vi "com VISA_atlas (sub VI).vi"(0 "Sensor":string(combo)="Temp", 1 "entrée d'erreur (pas d'erreur)":errorcluster) -> (2 "Output cluster":T1, 3 "Com found ?":bool)   [LabVIEW 2016]
doc: "Looks for the COM port corresponding to the necessary sensor. For Atlas sensor, sends a Information command (I \\r) and reads the response. Also determines the message size (in bytes) of a typical reading (with a 'R \\r' command)"
uses:
  Visa com cluster def (subVI).ctl
  <vilib>/Instr/_visa.llb/VISA Find Search Mode.ctl
  <vilib>/Instr/_visa.llb/VISA Set IO Buffer Mask.ctl
  <vilib>/Instr/_visa.llb/VISA Flush IO Buffer Mask.ctl
  <vilib>/Instr/_visa.llb/VISA Configure Serial Port (Instr).vi
  <vilib>/regexp/Match Regular Expression.xnode
panel:
  out "Reponse VISA":string
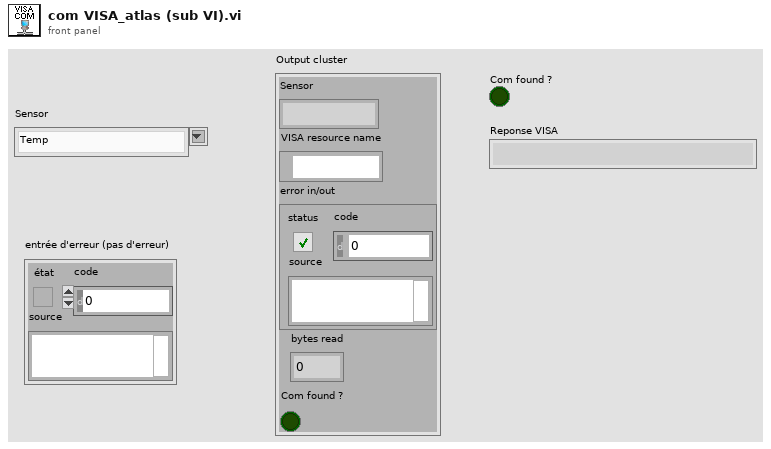
[diagram p1: front panel]
types:
  T1 = typedef "Visa com cluster def (subVI).ctl" = cluster{"Sensor":string, "VISA resource name":refnum<visa-resource-name>, "error in/out":errorcluster, "bytes read":u32, "Com found ?":bool}
  T2 = typedef "VISA Find Search Mode.ctl" = u32
  T3 = cluster{"baud rate":u32, "data bits":u16, "parity":enum16{"None", "Odd", "Even", "Mark", "Space"}, "stop bits":u16, "flow control":u16}
  T4 = typedef "VISA Flush IO Buffer Mask.ctl" = u16
  T5 = typedef "VISA Set IO Buffer Mask.ctl" = u16
  T6 = cluster{"Sensor":string, "VISA resource name out":refnum<visa-resource-name>, "error out":errorcluster, "bytes read":u32, bool}
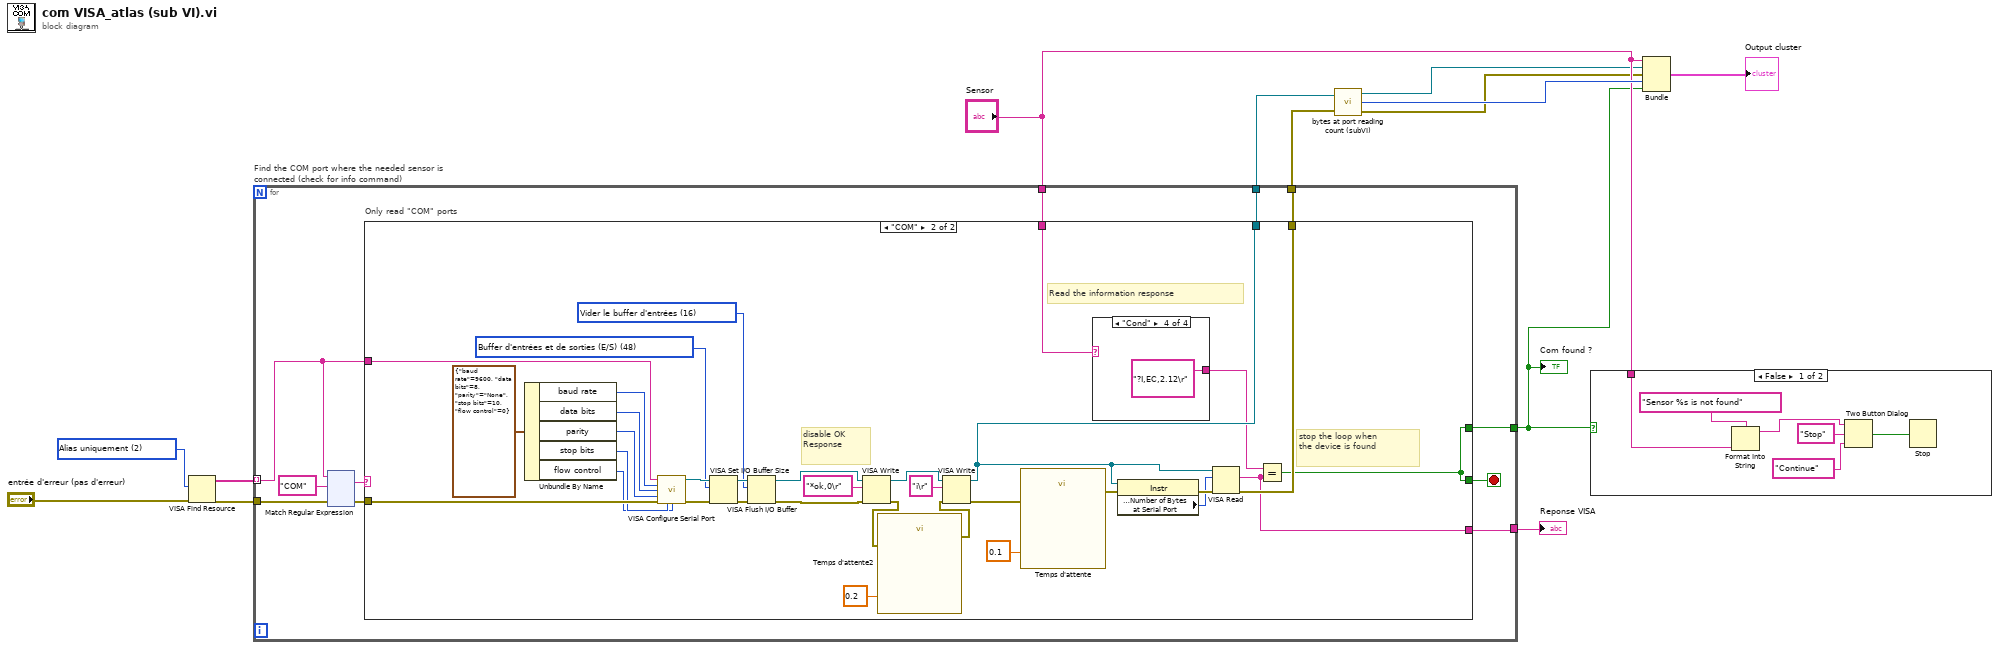
[diagram p0: block diagram]
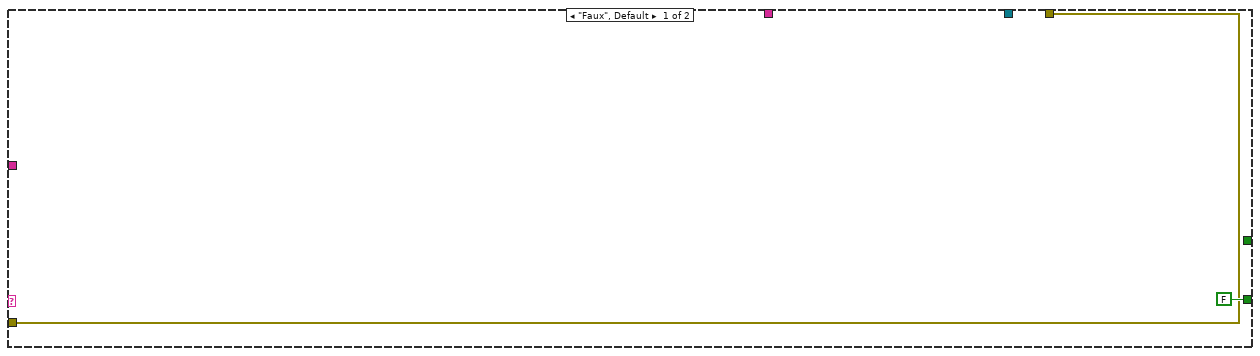
[diagram p3: hidden frame]
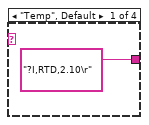
[diagram p4: hidden frame]
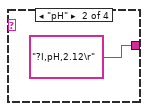
[diagram p5: hidden frame]
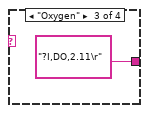
[diagram p6: hidden frame]
diagram:
  w10 = T2 2 items=["Noms canoniques uniquement"=0, "Alias uniquement"=2, "Inclure les alias correspondants"=3, "Inclure tous les alias"=4] ("Search Mode")
  n1 = VISA Find Resource(8:"entrée d'erreur (pas d'erreur)", 10:w10) -> (0:w13:errorcluster, 3:w11:string[])  [unwired: 1 in, 1 out]
  n2 = for "Find the COM port where the needed sensor is connected (check for info command)" {
    tunnel: w11 -> [w22] mode=indexing
    tunnel: [w20] -> w7
    tunnel: [w19] -> w9
    tunnel: [w18] -> w4
    tunnel: w13 -> [w17]
    tunnel: [w15] -> w8
    tunnel: "Sensor" -> [w14]
    stop <- w21 stop-if-true
    n3 = xnode "Match Regular Expression"("chaîne en entrée"=w22, "expression régulière"="COM", "entrée d'erreur"=w17) -> ("toute l'expression"=w23:string, "sortie d'erreur"=w16:errorcluster)  [unwired: 3 in, 3 out]
    n4 = case "Only read \"COM\" ports" shown="\"COM\"" w23 {
      tunnel: w22 -> [_ w50]
      tunnel: [FALSE w47] -> w21
      tunnel: [w25 w49] -> w20
      tunnel: [_ w48] -> w19
      tunnel: [_ w47] -> w18
      tunnel: w16 -> [w25 w46]
      tunnel: [_ w45] -> w15
      tunnel: w14 -> [_ w27]
      frame "Faux", Default {
      }
      frame "COM" {
        w42 = T4 16 items=["Vider le buffer d'entrées"=16, "Écrire le buffer de sorties sur le périphérique"=32, "Vider le buffer d'entrées (Pas d'E/S)"=64, "Vider le buffer de sorties"=128] ("Mask")
        w57 = T5 48 items=["Buffer d'entrées (E/S)"=16, "Buffer de sorties (E/S)"=32, "Buffer d'entrées et de sorties (E/S)"=48] ("Mask")
        # "disable OK\nResponse"
        # "Read the information response"
        # "stop the loop when \nthe device is found"
        n5 = Unbundle By Name(T3 {"baud rate"=9600, "data bits"=8, "parity"=enum."None", "stop bits"=10, "flow control"=0} ("Serial Settings")) -> ("baud rate"=w40:u32, "data bits"=w39:u16, "parity"=w38:enum16{"None", "Odd", "Even", "Mark", "Space"}, "stop bits"=w37:u16, "flow control"=w36:u16)
        n6 = call-poly "VISA Configure Serial Port"("VISA resource name"=w50, "baud rate (9600)"=w40, "data bits (8)"=w39, "parity (0:none)"=w38, "error in (no error)"=w46, "stop bits (10: 1 bit)"=w37, "flow control (0:none)"=w36) -> ("VISA resource name out"=w58:refnum<visa-resource-name>, "error out"=w59:errorcluster)  [unwired: 7 in]
        n7 = VISA Set I/O Buffer Size(VISA resource name=w58, mask (16)=w57, error in (no error)=w59) -> (VISA resource name out=w44:refnum<visa-resource-name>, error out=w43:errorcluster)  [unwired: 1 in]
        n8 = VISA Flush I/O Buffer(VISA resource name=w44, mask (16)=w42, error in (no error)=w43) -> (VISA resource name out=w32:refnum<visa-resource-name>, error out=w33:errorcluster)
        n9 = VISA Write(VISA resource name=w32, write buffer="*ok,0\r" ("buffer d'écriture"), error in (no error)=w33) -> (VISA resource name out=w31:refnum<visa-resource-name>, error out=w29:errorcluster)  [unwired: 1 out]
        n10 = call "Temps d'attente2"("error in (no error)"=w29, "Delay Time (s)"=0.2) -> ("error out"=w28:errorcluster)  [unwired: 9 in]
        n11 = VISA Write(VISA resource name=w31, write buffer="i\r" ("buffer d'écriture"), error in (no error)=w28) -> (VISA resource name out=w45:refnum<visa-resource-name>, error out=w55:errorcluster)  [unwired: 1 out]
        n12 = call "Temps d'attente"("error in (no error)"=w55, "Delay Time (s)"=0.1) -> ("error out"=w54:errorcluster)  [unwired: 9 in]
        n13 = case shown="\"Cond\"" w27 {
          tunnel: ["?I,RTD,2.10\r" ("Response 2") "?I,pH,2.12\r" ("Response 2") "?I,DO,2.11\r" ("Response 2") "?I,EC,2.12\r" ("Response 2")] -> w35
          frame "Temp", Default {
          }
          frame "pH" {
          }
          frame "Oxygen" {
          }
          frame "Cond" {
          }
        }
        n14 = property class="Instr"(reference=w45, error in=w54) -> (error out=w53:errorcluster, "Serial Settings:Number of Bytes at Serial Port"=w52:u32)  [unwired: 1 out]
        n15 = VISA Read(VISA resource name=w45, byte count=w52, error in (no error)=w53) -> (read buffer=w48:string, error out=w49:errorcluster)  [unwired: 2 out]
        n16 = Equal?(x=w35, y=w48) -> (x = y?=w47:bool)
      }
    }
  }
  "Reponse VISA" <- w9
  "Com found ?" <- w4
  n17 = call "bytes at port reading count (subVI).vi"("VISA Refnum in"=w8, "error in (no error)"=w7) -> ("VISA resource name out"=w1:refnum<visa-resource-name>, "bytes read"=w6:u32, "error out"=w2:errorcluster)
  n18 = case shown="False" w4 {
    tunnel: "Sensor" -> [w176 _]
    frame False {
      n19 = Format Into String(format string="Sensor %s is not found" ("error source (\" \")"), w176) -> (resulting string=w175:string)  [unwired: 2 in, 1 out]
      n20 = Two Button Dialog(message=w175, 1:"Continue" ("F button name (\"Cancel\")"), 2:"Stop" ("T button name (\"OK\")")) -> (T button?=w178:bool)
      n21 = Stop(stop? (T)=w178) -> ()
    }
    frame True {
    }
  }
  n22 = Bundle("Sensor"="Sensor", "VISA resource name out"=w1, "error out"=w2, "bytes read"=w6, w4) -> (→"Output cluster":T6)  [unwired: 1 in]
